vi "Helper SubVI - PWVD Kernel.vi"(8 "error in (no error)":errorcluster, 9 "alpha":dbl=1e-06, 10 "num of frequency bins":i32=-1, 11 "length":i32) -> (0 "error out":errorcluster, 1 "kernel":dbl[][](array[numeric]))   [LabVIEW 2023]
doc: "Gets the Pseudo Wigner-Ville Distribution (PWVD) kernel."
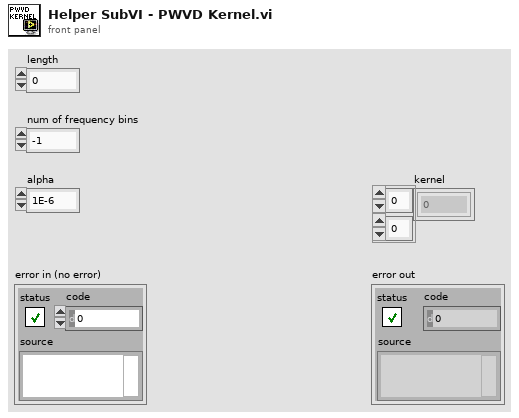
[diagram p1: front panel]
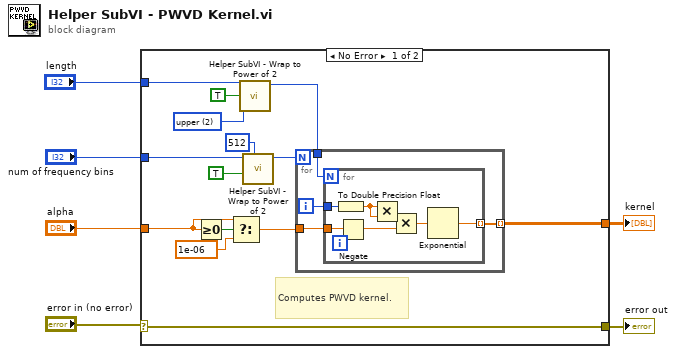
[diagram p0: block diagram]
diagram:
  n1 = case shown="No Error" "error in (no error)" {
    selector: "error in (no error)" -> [w7 w32]
    tunnel: [w13 _] -> w6
    tunnel: "num of frequency bins" -> [w17 _]
    tunnel: [w7 w32] -> w3
    tunnel: "alpha" -> [w10 _]
    tunnel: "length" -> [w12 _]
    frame No Error {
      w18 = u16 2 items=["nearest", "lower", "upper"] ("where to go")
      # "Computes PWVD kernel."
      n2 = Greater Or Equal To 0?(x=w10) -> (x >= 0?=w8:bool)
      n3 = Select(t=w10, s=w8, f=1e-06) -> (s? t:f=w9:dbl)
      n4 = call "Helper SubVI - Wrap to Power of 2.vi"("where to go"=w18, "power of 2"=TRUE, "number in"=w12) -> ("number out"=w15:i32)  [unwired: 8 in]
      n5 = call "Helper SubVI - Wrap to Power of 2.vi"("default"=512, "power of 2"=TRUE, "number in"=w17) -> ("number out"=w14:i32)  [unwired: 8 in]
      n6 = for {
        N: w14 -> [_]
        tunnel: w9 -> [w24]
        tunnel: [w23] -> w13 mode=indexing
        tunnel: w15 -> [w21]
        i -> [w22]
        n7 = for {
          N: w21 -> [_]
          tunnel: w24 -> [w30]
          tunnel: [w31] -> w23 mode=indexing
          tunnel: w22 -> [w29]
          n8 = To Double Precision Float(number=w29) -> (double precision float=w28:dbl)
          n9 = Negate(x=w30) -> (-x=w26:dbl)
          n10 = Multiply(x=w28, y=w28) -> (x*y=w27:dbl)
          n11 = Multiply(x=w27, y=w26) -> (x*y=w25:dbl)
          n12 = Exponential(1:w25) -> (0:w31:dbl)
        }
      }
    }
    frame Error {
    }
  }
  "kernel" <- w6
  "error out" <- w3
